vi "LSMcontroller_v58.vi"() -> ()   [LabVIEW 2015] (continued)
                    n4765 = Index Array(array=w1624, index=w1622) -> (element=w1623:T18)
                    n4766 = call "waveformsAObuffer.vi"("command"="get") -> ("AO wf out"=w1629:waveform(dbl)[])  [unwired: 1 in]
                    n4767 = call "matlabAOwffromparam.vi"("Cluster"=w1623) -> ("Waveform"=w1627:waveform(dbl))  [unwired: 1 out]
                    n4768 = property on="refwf" class="Ring (strict)"() -> ("RingText.Text"=w1630:string)  [unwired: 2 in, 2 out]
                    n4769 = Replace Array Subset(array=w1629, new element=w1627, index=w1622) -> (w1628:waveform(dbl)[])
                    n4770 = call "waveformsDObuffer.vi"("command"="get") -> ("DO wf out"=w1635:digitalwaveform[])  [unwired: 1 in]
                    n4771 = call "correctwaveformsizetemp.vi"("new sampling frequency (Hz)"=w1618, "start"=FALSE, "reference waveforms to"=w1630, "Analog waveforms in"=w1628, "stop"=FALSE, "Digital waveforms in"=w1635) -> ("analog wf out"=w1633:waveform(dbl)[], "Digital wf out"=w1631:digitalwaveform[], "measpoints"=w1620:i32)
                    n4772 = local read "wavdet"() -> (w1621:bool)
                    n4773 = local write "Analog Lines Plot"(w1633) -> ()
                    n4774 = call "GetNumCamFramesv2.vi"("Digital Waveform Graph"=w1631) -> ("Numeric"=w1632:i32)  [unwired: 10 in]
                    n4775 = local write "Digital Lines Plot"(w1631) -> ()
                    n4776 = call "waveformsAObuffer.vi"("AO wf in"=w1633, "command"="set") -> ()  [unwired: 1 out]
                    n4777 = call "waveformsDObuffer.vi"("DO wf in"=w1631, "command"="set") -> ()  [unwired: 1 out]
                    n4778 = local write "Total Camera Frames"(w1632) -> ()
                    n4779 = case shown="True" w1621 {
                      tunnel: w1620 -> [_ w1641]
                      frame False {
                      }
                      frame True {
                        n4780 = local write "# of frames"(w1641) -> ()
                      }
                    }
                  }
                }
              }
              frame #4 {
                n4781 = local read "finite samples"() -> (w1642:bool)
                n4782 = local read "continuous"() -> (w1643:bool)
                n4783 = local read "wavdet"() -> (w1644:bool)
                n4784 = call "2pparameters.vi"("command"="get") -> ("params out"=w1647:T12)  [unwired: 1 in]
                n4785 = Bundle By Name(cluster=w1647, "finite"=w1642, "cont"=w1643, "wavdet"=w1644) -> (w1645:T12)
                n4786 = call "2pparameters.vi"("Params in"=w1645, "command"="set") -> ()  [unwired: 1 out]
              }
            }
          }
          event "Load Matlab Waveform DO": Value Change {
            n4787 = event-data() -> ()  [unwired: 1 in, 6 out]
            n4788 = stacked-sequence {
              seq-local: [_ _ w1755 _ _] -> [_ _ _ w1770 _]
              seq-local: [_ _ w1754 _ _] -> [_ _ _ w1769 _]
              frame #0 {
                n4789 = local read "Measurement"() -> (w1649:T5)
                n4790 = case shown="\"X-Y-t movie\", Default" w1649 {
                  frame "X-Y-t movie", Default {
                    n4791 = local read "avpp"() -> (w1670:i32)
                    n4792 = local read "Angle ref"() -> (w1669:dbl)
                    n4793 = local read "ROI Type"() -> (w1668:u16)
                    n4794 = local read "xpixels ref"() -> (w1665:i32)
                    n4795 = local read "Vx-min ref"() -> (w1664:dbl)
                    n4796 = local read "Vx-max ref"() -> (w1663:dbl)
                    n4797 = local read "ypixels ref"() -> (w1661:i32)
                    n4798 = local read "Vy-min ref"() -> (w1662:dbl)
                    n4799 = local read "Vy-max ref"() -> (w1658:dbl)
                    n4800 = local read "Sampling rate"() -> (w1652:dbl)
                    n4801 = local read "finite samples"() -> (w1653:bool)
                    n4802 = local read "continuous"() -> (w1656:bool)
                    n4803 = local read "wavdet"() -> (w1657:bool)
                    n4804 = local read "# of frames"() -> (w1655:i32)
                    n4805 = local read "maxbufferAI"() -> (w1654:i32)
                    n4806 = local read "Override AI buffer"() -> (w1650:bool)
                    n4807 = call "2pparameters.vi"("command"="get") -> ("params out"=w1667:T12)  [unwired: 1 in]
                    n4808 = Bundle By Name(cluster=w1667, "type"="X-Y-t movie", "avpp"=w1670, "Angle Img"=w1669, "Xpixels Img"=w1665, "Vx-min Img"=w1664, "VX-max Img"=w1663, "Ypixels Img"=w1661, "Vy-min Img"=w1662, "Vy-max Img"=w1658, "srate"=w1652, "srate Img"=w1652, "finite"=w1653, "cont"=w1656, "wavdet"=w1657, "measpoints"=w1655, "maxbufferAI"=w1654, "Drawing Mode"=w1668, "Vz-reset"=0.0, "AIoverride"=w1650) -> (w1659:T12)
                    n4809 = call "2pparameters.vi"("Params in"=w1659, "command"="set") -> ()  [unwired: 1 out]
                  }
                  frame "X-Y-Z stack" {
                    n4810 = call "2pparameters.vi"("command"="get") -> ("params out"=w1674:T12)  [unwired: 1 in]
                    n4811 = Bundle By Name(cluster=w1674, "type"="X-Y-Z stack") -> (w1672:T12)
                    n4812 = call "2pparameters.vi"("Params in"=w1672, "command"="set") -> ()  [unwired: 1 out]
                  }
                  frame "Lifetime (scan)" {
                    n4813 = call "2pparameters.vi"("command"="get") -> ("params out"=w1679:T12)  [unwired: 1 in]
                    n4814 = Bundle By Name(cluster=w1679, "type"="Lifetime (scan)") -> (w1677:T12)
                    n4815 = call "2pparameters.vi"("Params in"=w1677, "command"="set") -> ()  [unwired: 1 out]
                  }
                  frame "Lifetime (contour)" {
                    n4816 = local read "Vy-min draw"() -> (w1689:dbl)
                    n4817 = local read "Vy-max draw"() -> (w1688:dbl)
                    n4818 = local read "Vx-min draw"() -> (w1691:dbl)
                    n4819 = local read "Vx-max draw"() -> (w1690:dbl)
                    n4820 = local read "xpixels ref"() -> (w1687:i32)
                    n4821 = local read "ypixels ref"() -> (w1686:i32)
                    n4822 = local read "ROI Type"() -> (w1685:u16)
                    n4823 = local read "srateAODOtt"() -> (w1696:dbl)
                    n4824 = local read "# of frames"() -> (w1701:i32)
                    n4825 = local read "refreshtime"() -> (w1693:dbl)
                    n4826 = local read "Pel"() -> (w1684:dbl)
                    n4827 = local read "bin"() -> (w1699:dbl)
                    n4828 = local read "Override AI buffer"() -> (w1682:bool)
                    n4829 = local read "finite samples"() -> (w1708:bool)
                    n4830 = local read "srateAODOtt"() -> (w1695:dbl)
                    n4831 = local read "srateAODOtt"() -> (w1702:dbl)
                    n4832 = local read "continuous"() -> (w1707:bool)
                    n4833 = local read "Angle ref"() -> (w1692:dbl)
                    n4834 = local read "wavdet"() -> (w1709:bool)
                    n4835 = local read "Vx-ref"() -> (w1704:dbl)
                    n4836 = local read "Vy-ref"() -> (w1706:dbl)
                    n4837 = local read "avpp"() -> (w1705:i32)
                    n4838 = call "tt_timeandsamples.vi"("bin"=w1699, "refreshtime"=w1693, "srateAODOtt"=w1696, "tot#ofsamples"=w1701) -> ("refreshrate"=w1697:dbl, "refreshbuffer"=w1698:i32, "timetracecycles"=w1703:i32)  [unwired: 5 in]
                    n4839 = local read "bin"() -> (w1700:dbl)
                    n4840 = call "2pparameters.vi"("command"="get") -> ("params out"=w1712:T12)  [unwired: 1 in]
                    n4841 = Bundle By Name(cluster=w1712, "Drawing Mode"=w1685, "measpoints"=w1701, "tt_cycles"=w1703, "refreshbuffer"=w1698, "refreshrate"=w1697, "Vx-ref"=w1704, "Vy-ref"=w1706, "srate"=w1695, "finite"=w1708, "cont"=w1707, "wavdet"=w1709, "avpp"=w1705, "srateAODO"=w1702, "bufferAI"=w1698, "bin"=w1700, "Angle Img"=w1692, "Vxminref"=w1691, "Vxmaxref"=w1690, "Vyminref"=w1689, "Vymaxref"=w1688, "Xpixels Img"=w1687, "Ypixels Img"=w1686, "Pel"=w1684, "Vz-reset"=0.0, "AIoverride"=w1682, "type"="Lifetime (contour)") -> (w1710:T12)
                    n4842 = Reciprocal(x=w1697) -> (1/x=w1694:dbl)
                    n4843 = local write "refreshtime"(w1694) -> ()
                    n4844 = call "2pparameters.vi"("Params in"=w1710, "command"="set") -> ()  [unwired: 1 out]
                  }
                  frame "X-Y-Z-t movie" {
                  }
                  frame "linescan" {
                  }
                  frame "Timetrace" {
                    n4845 = local read "Vy-min draw"() -> (w1722:dbl)
                    n4846 = local read "Vy-max draw"() -> (w1721:dbl)
                    n4847 = local read "Vx-min draw"() -> (w1724:dbl)
                    n4848 = local read "Vx-max draw"() -> (w1723:dbl)
                    n4849 = local read "xpixels ref"() -> (w1720:i32)
                    n4850 = local read "ypixels ref"() -> (w1719:i32)
                    n4851 = local read "ROI Type"() -> (w1718:u16)
                    n4852 = local read "srateAODOtt"() -> (w1729:dbl)
                    n4853 = local read "# of frames"() -> (w1734:i32)
                    n4854 = local read "refreshtime"() -> (w1726:dbl)
                    n4855 = local read "Pel"() -> (w1717:dbl)
                    n4856 = local read "bin"() -> (w1732:dbl)
                    n4857 = local read "Override AI buffer"() -> (w1715:bool)
                    n4858 = local read "finite samples"() -> (w1741:bool)
                    n4859 = local read "srateAODOtt"() -> (w1728:dbl)
                    n4860 = local read "srateAODOtt"() -> (w1735:dbl)
                    n4861 = local read "continuous"() -> (w1740:bool)
                    n4862 = local read "Angle ref"() -> (w1725:dbl)
                    n4863 = local read "wavdet"() -> (w1742:bool)
                    n4864 = local read "Vx-ref"() -> (w1737:dbl)
                    n4865 = local read "Vy-ref"() -> (w1739:dbl)
                    n4866 = local read "avpp"() -> (w1738:i32)
                    n4867 = call "tt_timeandsamples.vi"("bin"=w1732, "refreshtime"=w1726, "srateAODOtt"=w1729, "tot#ofsamples"=w1734) -> ("refreshrate"=w1730:dbl, "refreshbuffer"=w1731:i32, "timetracecycles"=w1736:i32)  [unwired: 5 in]
                    n4868 = local read "bin"() -> (w1733:dbl)
                    n4869 = call "2pparameters.vi"("command"="get") -> ("params out"=w1745:T12)  [unwired: 1 in]
                    n4870 = Bundle By Name(cluster=w1745, "Drawing Mode"=w1718, "measpoints"=w1734, "tt_cycles"=w1736, "refreshbuffer"=w1731, "refreshrate"=w1730, "Vx-ref"=w1737, "Vy-ref"=w1739, "srate"=w1728, "finite"=w1741, "cont"=w1740, "wavdet"=w1742, "avpp"=w1738, "srateAODO"=w1735, "bufferAI"=w1731, "bin"=w1733, "Angle Img"=w1725, "Vxminref"=w1724, "Vxmaxref"=w1723, "Vyminref"=w1722, "Vymaxref"=w1721, "Xpixels Img"=w1720, "Ypixels Img"=w1719, "Pel"=w1717, "Vz-reset"=0.0, "AIoverride"=w1715, "type"="Timetrace") -> (w1743:T12)
                    n4871 = Reciprocal(x=w1730) -> (1/x=w1727:dbl)
                    n4872 = local write "refreshtime"(w1727) -> ()
                    n4873 = call "2pparameters.vi"("Params in"=w1743, "command"="set") -> ()  [unwired: 1 out]
                  }
                  frame "Lifetime (point)" {
                  }
                }
              }
              frame #1 {
                w1748 = FALSE ("wavdet")
                n4874 = call "2pparameters.vi"("command"="get") -> ("params out"=w1752:T12)  [unwired: 1 in]
                n4875 = Bundle By Name(cluster=w1752, "finite"=w1748, "cont"=w1748, "wavdet"=TRUE) -> (w1749:T12)
                n4876 = call "2pparameters.vi"("Params in"=w1749, "command"="set") -> ()  [unwired: 1 out]
              }
              frame #2 {
                n4877 = local read "DO channels"() -> (w1757:u16)
                n4878 = call "2pparameters.vi"("command"="get") -> ("params out"=w1759:T12)  [unwired: 1 in]
                n4879 = Unbundle By Name(w1759) -> ("aDO"=w1758:u32[])
                n4880 = Search 1D Array(1D array=w1758, element=w1757) -> (index of element=w1755:i32)  [unwired: 1 in]
                n4881 = Greater?(x=w1755, y=-1) -> (0:w1754:bool)
                n4882 = case shown="True" w1754 {
                  tunnel: w1755 -> [_ w1766]
                  frame False {
                  }
                  frame True {
                    n4883 = local read "Meastab"() -> (w1762:enum32{"X-Y Image", "Linescan", "Timetrace"})
                    n4884 = local read "Matlab waveform path DO"() -> (w1764:path)
                    n4885 = local read "Matlab padding value DO"() -> (w1765:dbl)
                    n4886 = case shown="\"Timetrace\"" w1762 {
                      tunnel: [w1767 w1768] -> w1761
                      frame "X-Y Image", Default {
                        n4887 = local read "Sampling rate"() -> (w1767:dbl)
                      }
                      frame "Timetrace" {
                        n4888 = local read "srateAODOtt"() -> (w1768:dbl)
                      }
                    }
                    n4889 = call "matlabwfexistsdialogue.vi"("Matlab waveform path"=w1764) -> ("mtalab waveform path out"=w1763:path)
                    n4890 = call "replace DO matlab param.vi"("Sampling frequency (Hz)"=w1761, "matlab wave number"=w1763, "index of DO wave"=w1766, "padding value"=w1765) -> ()  [unwired: 7 in]
                  }
                }
              }
              frame #3 {
                n4891 = case shown="True" w1769 {
                  tunnel: w1770 -> [_ w1779]
                  frame False {
                  }
                  frame True {
                    n4892 = local read "Meastab"() -> (w1774:enum32{"X-Y Image", "Linescan", "Timetrace"})
                    n4893 = call "waveformparamsv2.vi"("command"="get") -> ("Params out"=w1792:T16)  [unwired: 4 in, 2 out]
                    n4894 = Unbundle By Name(w1792) -> ("DO parameters"=w1791:T19)
                    n4895 = case shown="\"Timetrace\"" w1774 {
                      tunnel: [w1794 w1795] -> w1773
                      frame "X-Y Image", Default {
                        n4896 = local read "Sampling rate"() -> (w1794:dbl)
                      }
                      frame "Timetrace" {
                        n4897 = local read "srateAODOtt"() -> (w1795:dbl)
                      }
                    }
                    n4898 = Index Array(array=w1791, index=w1779) -> (element=w1778:T20)
                    n4899 = call "waveformsDObuffer.vi"("command"="get") -> ("DO wf out"=w1789:digitalwaveform[])  [unwired: 1 in]
                    n4900 = property on="refwf" class="Ring (strict)"() -> ("RingText.Text"=w1781:string)  [unwired: 2 in, 2 out]
                    n4901 = call "matlabDOwffromparam.vi"("waveform params"=w1778) -> ("digital waveform"=w1777:digitalwaveform)
                    n4902 = Replace Array Subset(array=w1789, new element=w1777, index=w1779) -> (w1780:digitalwaveform[])
                    n4903 = call "waveformsAObuffer.vi"("command"="get") -> ("AO wf out"=w1788:waveform(dbl)[])  [unwired: 1 in]
                    n4904 = local read "wavdet"() -> (w1776:bool)
                    n4905 = call "correctwaveformsizetemp.vi"("new sampling frequency (Hz)"=w1773, "start"=FALSE, "reference waveforms to"=w1781, "Analog waveforms in"=w1788, "stop"=FALSE, "Digital waveforms in"=w1780) -> ("analog wf out"=w1784:waveform(dbl)[], "Digital wf out"=w1782:digitalwaveform[], "measpoints"=w1775:i32)
                    n4906 = local write "Analog Lines Plot"(w1784) -> ()
                    n4907 = call "GetNumCamFramesv2.vi"("Digital Waveform Graph"=w1782) -> ("Numeric"=w1783:i32)  [unwired: 10 in]
                    n4908 = local write "Digital Lines Plot"(w1782) -> ()
                    n4909 = case shown="True" w1776 {
                      tunnel: w1775 -> [_ w1796]
                      frame False {
                      }
                      frame True {
                        n4910 = local write "# of frames"(w1796) -> ()
                      }
                    }
                    n4911 = call "waveformsAObuffer.vi"("AO wf in"=w1784, "command"="set") -> ()  [unwired: 1 out]
                    n4912 = call "waveformsDObuffer.vi"("DO wf in"=w1782, "command"="set") -> ()  [unwired: 1 out]
                    n4913 = local write "Total Camera Frames"(w1783) -> ()
                  }
                }
              }
              frame #4 {
                n4914 = local read "finite samples"() -> (w1797:bool)
                n4915 = local read "continuous"() -> (w1798:bool)
                n4916 = local read "wavdet"() -> (w1799:bool)
                n4917 = call "2pparameters.vi"("command"="get") -> ("params out"=w1802:T12)  [unwired: 1 in]
                n4918 = Bundle By Name(cluster=w1802, "finite"=w1797, "cont"=w1798, "wavdet"=w1799) -> (w1800:T12)
                n4919 = call "2pparameters.vi"("Params in"=w1800, "command"="set") -> ()  [unwired: 1 out]
              }
            }
          }
          event "Add settings": Value Change {
            n4920 = event-data() -> ()  [unwired: 1 in, 6 out]
            n4921 = call "wfsettings.vi"("command"="get") -> ("wfsettings out"=w1806:T29)  [unwired: 2 in, 1 out]
            n4922 = in-place {
              n4923 = in-place-cluster #53(w1806) -> ("settings names"=w1811:string[], "settings locations"=w1813:path[])
              n4924 = local read "Setting location"() -> (w1809:path)
              n4925 = local read "Nickname"() -> (w1808:string)
              n4926 = Build Array (concatenate)(w1811, w1808) -> (w1810:string[])
              n4927 = property on="Loaded settings" class="Ring (strict)"("Strings []"=w1810) -> ()  [unwired: 2 in, 2 out]
              n4928 = Build Array (concatenate)(w1813, w1809) -> (w1812:path[])
              n4929 = in-place-cluster #53("settings names"=w1810, "settings locations"=w1812) -> (w1804:T29)
            }
            n4930 = call "wfsettings.vi"("wfsettings in"=w1804, "command"="set") -> ()  [unwired: 1 in, 2 out]
          }
          event "Rem setting": Value Change {
            n4931 = event-data() -> ()  [unwired: 1 in, 6 out]
            n4932 = call "wfsettings.vi"("command"="get") -> ("wfsettings out"=w1816:T29)  [unwired: 2 in, 1 out]
            n4933 = in-place {
              n4934 = in-place-cluster #54(w1816) -> ("settings names"=w1821:string[], "settings locations"=w1819:path[])
              n4935 = property on="Loaded settings" class="Ring (strict)"() -> ("RingText.Text"=w1822:string)  [unwired: 2 in, 2 out]
              n4936 = Search 1D Array(1D array=w1821, element=w1822) -> (index of element=w1823:i32)  [unwired: 1 in]
              n4937 = Delete From Array(array=w1821, index=w1823) -> (array with subset deleted=w1820:string[])  [unwired: 1 in, 1 out]
              n4938 = Delete From Array(array=w1819, index=w1823) -> (array with subset deleted=w1818:path[])  [unwired: 1 in, 1 out]
              n4939 = property on="Loaded settings" class="Ring (strict)"("Strings []"=w1820) -> ()  [unwired: 2 in, 2 out]
              n4940 = in-place-cluster #54("settings names"=w1820, "settings locations"=w1818) -> (w1814:T29)
            }
            n4941 = call "wfsettings.vi"("wfsettings in"=w1814, "command"="set") -> ()  [unwired: 1 in, 2 out]
          }
          event "Update settings": Value Change {
            n4942 = event-data() -> ()  [unwired: 1 in, 6 out]
            n4943 = stacked-sequence {
              frame #0 {
                n4944 = local read "Measurement"() -> (w1824:T5)
                n4945 = case shown="\"Timetrace\"" w1824 {
                  frame "X-Y-t movie", Default {
                    n4946 = local read "avpp"() -> (w1845:i32)
                    n4947 = local read "Angle ref"() -> (w1844:dbl)
                    n4948 = local read "ROI Type"() -> (w1843:u16)
                    n4949 = local read "xpixels ref"() -> (w1840:i32)
                    n4950 = local read "Vx-min ref"() -> (w1839:dbl)
                    n4951 = local read "Vx-max ref"() -> (w1838:dbl)
                    n4952 = local read "ypixels ref"() -> (w1836:i32)
                    n4953 = local read "Vy-min ref"() -> (w1837:dbl)
                    n4954 = local read "Vy-max ref"() -> (w1833:dbl)
                    n4955 = local read "Sampling rate"() -> (w1827:dbl)
                    n4956 = local read "finite samples"() -> (w1828:bool)
                    n4957 = local read "continuous"() -> (w1831:bool)
                    n4958 = local read "wavdet"() -> (w1832:bool)
                    n4959 = local read "# of frames"() -> (w1830:i32)
                    n4960 = local read "maxbufferAI"() -> (w1829:i32)
                    n4961 = local read "Override AI buffer"() -> (w1825:bool)
                    n4962 = call "2pparameters.vi"("command"="get") -> ("params out"=w1842:T12)  [unwired: 1 in]
                    n4963 = Bundle By Name(cluster=w1842, "type"="X-Y-t movie", "avpp"=w1845, "Angle Img"=w1844, "Xpixels Img"=w1840, "Vx-min Img"=w1839, "VX-max Img"=w1838, "Ypixels Img"=w1836, "Vy-min Img"=w1837, "Vy-max Img"=w1833, "srate"=w1827, "srate Img"=w1827, "finite"=w1828, "cont"=w1831, "wavdet"=w1832, "measpoints"=w1830, "maxbufferAI"=w1829, "Drawing Mode"=w1843, "Vz-reset"=0.0, "AIoverride"=w1825) -> (w1834:T12)
                    n4964 = call "2pparameters.vi"("Params in"=w1834, "command"="set") -> ()  [unwired: 1 out]
                  }
                  frame "X-Y-Z stack" {
                    n4965 = call "2pparameters.vi"("command"="get") -> ("params out"=w1849:T12)  [unwired: 1 in]
                    n4966 = Bundle By Name(cluster=w1849, "type"="X-Y-Z stack") -> (w1847:T12)
                    n4967 = call "2pparameters.vi"("Params in"=w1847, "command"="set") -> ()  [unwired: 1 out]
                  }
                  frame "Lifetime (scan)" {
                    n4968 = call "2pparameters.vi"("command"="get") -> ("params out"=w1854:T12)  [unwired: 1 in]
                    n4969 = Bundle By Name(cluster=w1854, "type"="Lifetime (scan)") -> (w1852:T12)
                    n4970 = call "2pparameters.vi"("Params in"=w1852, "command"="set") -> ()  [unwired: 1 out]
                  }
                  frame "Lifetime (contour)" {
                    n4971 = local read "Vy-min draw"() -> (w1864:dbl)
                    n4972 = local read "Vy-max draw"() -> (w1863:dbl)
                    n4973 = local read "Vx-min draw"() -> (w1866:dbl)
                    n4974 = local read "Vx-max draw"() -> (w1865:dbl)
                    n4975 = local read "xpixels ref"() -> (w1862:i32)
                    n4976 = local read "ypixels ref"() -> (w1861:i32)
                    n4977 = local read "ROI Type"() -> (w1860:u16)
                    n4978 = local read "srateAODOtt"() -> (w1871:dbl)
                    n4979 = local read "# of frames"() -> (w1876:i32)
                    n4980 = local read "refreshtime"() -> (w1868:dbl)
                    n4981 = local read "Pel"() -> (w1859:dbl)
                    n4982 = local read "bin"() -> (w1874:dbl)
                    n4983 = local read "Override AI buffer"() -> (w1857:bool)
                    n4984 = local read "finite samples"() -> (w1883:bool)
                    n4985 = local read "srateAODOtt"() -> (w1870:dbl)
                    n4986 = local read "srateAODOtt"() -> (w1877:dbl)
                    n4987 = local read "continuous"() -> (w1882:bool)
                    n4988 = local read "Angle ref"() -> (w1867:dbl)
                    n4989 = local read "wavdet"() -> (w1884:bool)
                    n4990 = local read "Vx-ref"() -> (w1879:dbl)
                    n4991 = local read "Vy-ref"() -> (w1881:dbl)
                    n4992 = local read "avpp"() -> (w1880:i32)
                    n4993 = call "tt_timeandsamples.vi"("bin"=w1874, "refreshtime"=w1868, "srateAODOtt"=w1871, "tot#ofsamples"=w1876) -> ("refreshrate"=w1872:dbl, "refreshbuffer"=w1873:i32, "timetracecycles"=w1878:i32)  [unwired: 5 in]
                    n4994 = local read "bin"() -> (w1875:dbl)
                    n4995 = call "2pparameters.vi"("command"="get") -> ("params out"=w1887:T12)  [unwired: 1 in]
                    n4996 = Bundle By Name(cluster=w1887, "Drawing Mode"=w1860, "measpoints"=w1876, "tt_cycles"=w1878, "refreshbuffer"=w1873, "refreshrate"=w1872, "Vx-ref"=w1879, "Vy-ref"=w1881, "srate"=w1870, "finite"=w1883, "cont"=w1882, "wavdet"=w1884, "avpp"=w1880, "srateAODO"=w1877, "bufferAI"=w1873, "bin"=w1875, "Angle Img"=w1867, "Vxminref"=w1866, "Vxmaxref"=w1865, "Vyminref"=w1864, "Vymaxref"=w1863, "Xpixels Img"=w1862, "Ypixels Img"=w1861, "Pel"=w1859, "Vz-reset"=0.0, "AIoverride"=w1857, "type"="Lifetime (contour)") -> (w1885:T12)
                    n4997 = Reciprocal(x=w1872) -> (1/x=w1869:dbl)
                    n4998 = local write "refreshtime"(w1869) -> ()
                    n4999 = call "2pparameters.vi"("Params in"=w1885, "command"="set") -> ()  [unwired: 1 out]
                  }
                  frame "X-Y-Z-t movie" {
                  }
                  frame "linescan" {
                  }
                  frame "Timetrace" {
                    n5000 = local read "Vy-min draw"() -> (w1897:dbl)
                    n5001 = local read "Vy-max draw"() -> (w1896:dbl)
                    n5002 = local read "Vx-min draw"() -> (w1899:dbl)
                    n5003 = local read "Vx-max draw"() -> (w1898:dbl)
                    n5004 = local read "xpixels ref"() -> (w1895:i32)
                    n5005 = local read "ypixels ref"() -> (w1894:i32)
                    n5006 = local read "ROI Type"() -> (w1893:u16)
                    n5007 = local read "srateAODOtt"() -> (w1904:dbl)
                    n5008 = local read "# of frames"() -> (w1909:i32)
                    n5009 = local read "refreshtime"() -> (w1901:dbl)
                    n5010 = local read "Pel"() -> (w1892:dbl)
                    n5011 = local read "bin"() -> (w1907:dbl)
                    n5012 = local read "Override AI buffer"() -> (w1890:bool)
                    n5013 = local read "finite samples"() -> (w1916:bool)
                    n5014 = local read "srateAODOtt"() -> (w1903:dbl)
                    n5015 = local read "srateAODOtt"() -> (w1910:dbl)
                    n5016 = local read "continuous"() -> (w1915:bool)
                    n5017 = local read "Angle ref"() -> (w1900:dbl)
                    n5018 = local read "wavdet"() -> (w1917:bool)
                    n5019 = local read "Vx-ref"() -> (w1912:dbl)
                    n5020 = local read "Vy-ref"() -> (w1914:dbl)
                    n5021 = local read "avpp"() -> (w1913:i32)
                    n5022 = call "tt_timeandsamples.vi"("bin"=w1907, "refreshtime"=w1901, "srateAODOtt"=w1904, "tot#ofsamples"=w1909) -> ("refreshrate"=w1905:dbl, "refreshbuffer"=w1906:i32, "timetracecycles"=w1911:i32)  [unwired: 5 in]
                    n5023 = local read "bin"() -> (w1908:dbl)
                    n5024 = call "2pparameters.vi"("command"="get") -> ("params out"=w1920:T12)  [unwired: 1 in]
                    n5025 = Bundle By Name(cluster=w1920, "Drawing Mode"=w1893, "measpoints"=w1909, "tt_cycles"=w1911, "refreshbuffer"=w1906, "refreshrate"=w1905, "Vx-ref"=w1912, "Vy-ref"=w1914, "srate"=w1903, "finite"=w1916, "cont"=w1915, "wavdet"=w1917, "avpp"=w1913, "srateAODO"=w1910, "bufferAI"=w1906, "bin"=w1908, "Angle Img"=w1900, "Vxminref"=w1899, "Vxmaxref"=w1898, "Vyminref"=w1897, "Vymaxref"=w1896, "Xpixels Img"=w1895, "Ypixels Img"=w1894, "Pel"=w1892, "Vz-reset"=0.0, "AIoverride"=w1890, "type"="Timetrace") -> (w1918:T12)
                    n5026 = Reciprocal(x=w1905) -> (1/x=w1902:dbl)
                    n5027 = local write "refreshtime"(w1902) -> ()
                    n5028 = call "2pparameters.vi"("Params in"=w1918, "command"="set") -> ()  [unwired: 1 out]
                  }
                  frame "Lifetime (point)" {
                  }
                }
              }
              frame #1 {
                w1923 = FALSE ("wavdet")
                n5029 = call "2pparameters.vi"("command"="get") -> ("params out"=w1927:T12)  [unwired: 1 in]
                n5030 = Bundle By Name(cluster=w1927, "finite"=w1923, "cont"=w1923, "wavdet"=TRUE) -> (w1924:T12)
                n5031 = call "2pparameters.vi"("Params in"=w1924, "command"="set") -> ()  [unwired: 1 out]
              }
              frame #2 {
                n5032 = property on="Loaded settings" class="Ring (strict)"() -> ("RingText.Text"=w1929:string)  [unwired: 2 in, 2 out]
                n5033 = control-ref of="Analog Lines Plot"() -> (w1931:refnum<vi>)
                n5034 = control-ref of="Digital Lines Plot"() -> (w1930:refnum<vi>)
                n5035 = call "Usedlinesfromsettingsfile.vi"("sertting"=w1929) -> ("used AO names"=w1935:string[], "used AO lines"=w1934:tag[], "used DO names"=w1933:string[], "used DO lines"=w1932:tag[])
                n5036 = call "loadAODOwfparamsfromsettingsfile.vi"("sertting"=w1929) -> ()
                n5037 = call "prepAOWaveplot.vi"("WaveformGraph in"=w1931, "Analog Used Names"=w1935) -> ()  [unwired: 1 in]
                n5038 = local write "Analog Used Names"(w1935) -> ()
                n5039 = local write "Analog Used Lines"(w1934) -> ()
                n5040 = call "prepDOWaveplot.vi"("DigitalGraph in"=w1930, "used DO names"=w1933) -> ()  [unwired: 1 in]
                n5041 = local write "Digital Used Names"(w1933) -> ()
                n5042 = local write "Digital Used Lines"(w1932) -> ()
              }
              frame #3 {
                n5043 = call "waveformparamsv2.vi"("command"="get") -> ("Params out"=w1952:T16)  [unwired: 4 in, 2 out]
                n5044 = Unbundle By Name(w1952) -> ("AO parameters"=w1953:T17, "DO parameters"=w1954:T19)
                n5045 = for {
                  tunnel: w1953 -> [w1973] mode=indexing
                  tunnel: [w1971] -> w1955 mode=indexing
                  tunnel: [w1970] -> w1940 mode=indexing
                  tunnel: [w1968] -> w1943 mode=indexing
                  i -> [w1972]
                  n5046 = Unbundle By Name(w1973) -> ("AOtab"=w1974:dbl)
                  n5047 = case shown="0, Default" w1974 {
                    tunnel: w1973 -> [_ w1985 w1987 w1989]
                    tunnel: [_ w1984 w1986 w1988] -> w1969
                    frame -1 {
                    }
                    frame 0, Default {
                      n5048 = call "generateRampedSquareWave_fromAOparameters.vi"("AO params"=w1985) -> ("Waveform"=w1984:waveform(dbl))  [unwired: 1 out]
                    }
                    frame 1 {
                      n5049 = call "generateTriWave_fromAOparameters.vi"("AO params"=w1987) -> ("Waveform"=w1986:waveform(dbl))  [unwired: 1 out]
                    }
                    frame 2 {
                      n5050 = call "matlabAOwffromparam.vi"("Cluster"=w1989) -> ("Waveform"=w1988:waveform(dbl))  [unwired: 1 out]
                    }
                  }
                  n5051 = case shown="0" w1972 {
                    tunnel: [w1979 -1] -> w1971
                    tunnel: [w1978 w1982] -> w1970
                    tunnel: w1969 -> [w1978 w1982]
                    tunnel: [w1975 -1.0] -> w1968
                    frame 0 {
                      n5052 = Unbundle By Name(w1978) -> ("dt"=w1977:dbl, "Y"=w1980:dbl[])
                      n5053 = Reciprocal(x=w1977) -> (1/x=w1976:dbl)
                      n5054 = Array Size(array=w1980) -> (size(s)=w1979:i32)
                      n5055 = Round To Nearest(number=w1976) -> (nearest integer value=w1975:dbl)
                    }
                    frame 1, Default {
                    }
                  }
                }
                n5056 = Index Array(array=w1955, index=0) -> (element=w1957:i32)
                n5057 = Index Array(array=w1943, index=0) -> (element=w1942:dbl)
                n5058 = for {
                  tunnel: w1954 -> [w1962] mode=indexing
                  tunnel: [w1960] -> w1941 mode=indexing
                  tunnel: w1957 -> [w1959]
                  n5059 = Unbundle By Name(w1962) -> ("DOtab"=w1961:dbl)
                  n5060 = case shown="0, Default" w1961 {
                    tunnel: w1962 -> [w1965 w1967]
                    tunnel: w1959 -> [w1964 _]
                    tunnel: [w1963 w1966] -> w1960
                    frame 0, Default {
                      n5061 = call "simple digital from wf params.vi"("waveform params"=w1965, "number of samples"=w1964) -> ("digital waveform"=w1963:digitalwaveform)
                    }
                    frame 1 {
                      n5062 = call "matlabDOwffromparam.vi"("waveform params"=w1967) -> ("digital waveform"=w1966:digitalwaveform)
                    }
                  }
                }
                n5063 = property on="refwf" class="Ring (strict)"() -> ("RingText.Text"=w1945:string)  [unwired: 2 in, 2 out]
                n5064 = call "correctwaveformsizetemp.vi"("new sampling frequency (Hz)"=w1942, "start"=FALSE, "reference waveforms to"=w1945, "Analog waveforms in"=w1940, "stop"=FALSE, "Digital waveforms in"=w1941) -> ("analog wf out"=w1939:waveform(dbl)[], "Digital wf out"=w1938:digitalwaveform[], "measpoints"=w1936:i32)
                n5065 = local read "wavdet"() -> (w1937:bool)
                n5066 = case shown="True" w1937 {
                  tunnel: w1936 -> [_ w1958]
                  frame False {
                  }
                  frame True {
                    n5067 = local write "# of frames"(w1958) -> ()
                  }
                }
                n5068 = local write "Analog Lines Plot"(w1939) -> ()
                n5069 = local write "Digital Lines Plot"(w1938) -> ()
                n5070 = call "GetNumCamFramesv2.vi"("Digital Waveform Graph"=w1938) -> ("Numeric"=w1950:i32)  [unwired: 10 in]
                n5071 = call "waveformsAObuffer.vi"("AO wf in"=w1939, "command"="set") -> ()  [unwired: 1 out]
                n5072 = call "waveformsDObuffer.vi"("DO wf in"=w1938, "command"="set") -> ()  [unwired: 1 out]
                n5073 = local write "Total Camera Frames"(w1950) -> ()
              }
              frame #4 {
                n5074 = local read "AO channels"() -> (w1990:u32)
                n5075 = call "2pparameters.vi"("command"="get") -> ("params out"=w1992:T12)  [unwired: 1 in]
                n5076 = Unbundle By Name(w1992) -> ("aAO"=w1991:u32[])
                n5077 = Search 1D Array(1D array=w1991, element=w1990) -> (index of element=w1994:i32)  [unwired: 1 in]
                n5078 = Equal?(x=w1994, y=-1.0) -> (x = y?=w1995:bool)
                n5079 = case shown="False" w1995 {
                  tunnel: w1994 -> [w2020 _]
                  frame False {
                    n5080 = call "waveformparamsv2.vi"("command"="get") -> ("Params out"=w2003:T16)  [unwired: 4 in, 2 out]
                    n5081 = Unbundle By Name(w2003) -> ("AO parameters"=w2002:T17)
                    n5082 = Index Array(array=w2002, index=w2020) -> (element=w2019:T18)
                    n5083 = Unbundle By Name(w2019) -> ("AOtab"=w2000:dbl, "Repeats"=w2018:dbl, "Cycles"=w2017:dbl, "Start amplitude (V)"=w2016:dbl, "Baseline (V)"=w2015:dbl, "Step size (V)"=w2014:dbl, "DC (%)"=w2013:dbl, "Sampling frequency (Hz)"=w2012:dbl, "Period (ms)"=w2011:dbl, "Offset (V)"=w2010:dbl, "Amplitude (V)"=w2009:dbl, "Frequency"=w2008:dbl, "Tri Repeats"=w2007:dbl, "phase shift (ms)"=w2006:dbl, "Pulses"=w2005:dbl, "Tri phase"=w2001:dbl, "padding value"=w1997:dbl, "Matlab wave file"=w1998:path)
                    n5084 = To Unsigned Long Integer(number=w2000) -> (unsigned 32bit integer=w1999:u32)
                    n5085 = local write "Build analog waveform tabs"(w1999) -> ()
                    n5086 = local write "Matlab waveform path"(w1998) -> ()
                    n5087 = local write "phase shift (ms)"(w2006) -> ()
                    n5088 = local write "Repeats"(w2018) -> ()
                    n5089 = local write "Cycles"(w2017) -> ()
                    n5090 = local write "Amplitude (V)"(w2009) -> ()
                    n5091 = local write "Matlab padding value"(w1997) -> ()
                    n5092 = local write "Tri padding value"(w1997) -> ()
                    n5093 = local write "Start amplitude (V)"(w2016) -> ()
                    n5094 = local write "Tri Phase (s)"(w2001) -> ()
                    n5095 = local write "Period (ms)"(w2011) -> ()
                    n5096 = local write "Tri Repeats"(w2007) -> ()
                    n5097 = local write "Offset (V)"(w2010) -> ()
                    n5098 = local write "Frequency"(w2008) -> ()
                    n5099 = local write "Pulses"(w2005) -> ()
                    n5100 = local write "padding value"(w1997) -> ()
                    n5101 = local write "Sampling rate \ncurrent wf"(w2012) -> ()
                    n5102 = local write "Baseline (V)"(w2015) -> ()
                    n5103 = local write "Step size (V)"(w2014) -> ()
                    n5104 = local write "DC (%)"(w2013) -> ()
                  }
                  frame True {
                  }
                }
              }
              frame #5 {
                n5105 = local read "DO channels"() -> (w2023:u16)
                n5106 = call "2pparameters.vi"("command"="get") -> ("params out"=w2025:T12)  [unwired: 1 in]
                n5107 = Unbundle By Name(w2025) -> ("aDO"=w2024:u32[])
                n5108 = Search 1D Array(1D array=w2024, element=w2023) -> (index of element=w2022:i32)  [unwired: 1 in]
                n5109 = Equal?(x=w2022, y=-1.0) -> (x = y?=w2021:bool)
                n5110 = case shown="False" w2021 {
                  tunnel: w2022 -> [w2040 _]
                  frame False {
                    n5111 = call "waveformparamsv2.vi"("command"="get") -> ("Params out"=w2034:T16)  [unwired: 4 in, 2 out]
                    n5112 = Unbundle By Name(w2034) -> ("DO parameters"=w2032:T19)
                    n5113 = Index Array(array=w2032, index=w2040) -> (element=w2039:T20)
                    n5114 = Unbundle By Name(w2039) -> ("Digital DC (%)"=w2038:dbl, "Digital phase"=w2037:dbl, "Digital Freq (Hz)"=w2036:dbl, "Sampling frequency (Hz)"=w2035:dbl, "Digital time offset (s)"=w2031:dbl, "padding value"=w2030:dbl, "matlab wave file"=w2029:path, "DOtab"=w2028:dbl)
                    n5115 = local write "Build digital waveform tabs"(w2028) -> ()
                    n5116 = local write "Digital DC (%)"(w2038) -> ()
                    n5117 = local write "Matlab waveform path DO"(w2029) -> ()
                    n5118 = local write "Sampling rate \ncurrent wf"(w2035) -> ()
                    n5119 = local write "Digital time offset (s)"(w2031) -> ()
                    n5120 = local write "Matlab padding value DO"(w2030) -> ()
                    n5121 = local write "Digital padding value"(w2030) -> ()
                    n5122 = local write "Digital Freq (Hz)"(w2036) -> ()
                    n5123 = local write "Digital phase (s)"(w2037) -> ()
                  }
                  frame True {
                  }
                }
              }
              frame #6 {
                n5124 = local read "finite samples"() -> (w2041:bool)
                n5125 = local read "continuous"() -> (w2042:bool)
                n5126 = local read "wavdet"() -> (w2043:bool)
                n5127 = call "2pparameters.vi"("command"="get") -> ("params out"=w2046:T12)  [unwired: 1 in]
                n5128 = Bundle By Name(cluster=w2046, "finite"=w2041, "cont"=w2042, "wavdet"=w2043) -> (w2044:T12)
                n5129 = call "2pparameters.vi"("Params in"=w2044, "command"="set") -> ()  [unwired: 1 out]
              }
            }
          }
          event "Exit": Value Change {
            n5130 = event-data() -> ("NewVal"=w2048:bool)  [unwired: 1 in]
          }
        }
        n5131 = Wait (ms)(milliseconds to wait=u32 50) -> ()  [unwired: 1 out]
      }
    }
    frame #3 {
      w6615 = FALSE ("Value (Signaling)")
      n5132 = property on="Start" class="Bool (strict)"("Val(Sgnl)"=w6615) -> ()  [unwired: 2 in, 2 out]
      n5133 = property on="Exit" class="Bool (strict)"("Val(Sgnl)"=w6615) -> ()  [unwired: 2 in, 2 out]
      n5134 = property on="Stop" class="Bool (strict)"("Val(Sgnl)"=w6615) -> ()  [unwired: 2 in, 2 out]
      n5135 = flat-sequence {
        frame #0 {
          w6616 = u16 1 items=["OD 0"=1, "OD 0.5"=2, "OD 1"=3, "OD 2"=4, "OD 3"=5, "OD 4"=6] ("New ODfilt")
          n5136 = local read "ODfilt"() -> (w6617:u16)
          n5137 = call "filterwheelcontrol_nothorlabslib.vi"("Current OD filt"=w6617, "New ODfilt"=w6616) -> ()  [unwired: 1 in]
        }
        frame #1 {
          n5138 = Wait (ms)(milliseconds to wait=u32 1000) -> ()  [unwired: 1 out]
        }
      }
    }
  }
